vi "RSNRPZ Get Sensor Count.vi"(8 "error in (no error)":errorcluster) -> (0 "error out":errorcluster, 2 "Sensors Count":i32)   [LabVIEW 2010]
doc: "This VI returns the number of currently connected sensors."
uses:
  rsnrpz_32.dll
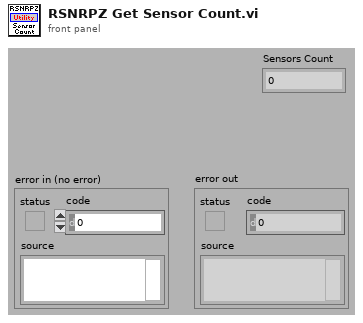
[diagram p1: front panel]
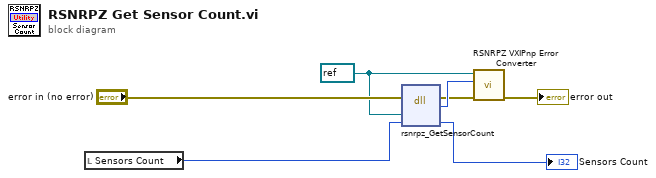
[diagram p0: block diagram]
diagram:
  w1 = refnum<visa-resource-name> refnum ("VISA session")
  n1 = local read "Sensors Count"() -> (w6:i32)
  n2 = dll-call lib="rsnrpz_32.dll" fn="rsnrpz_GetSensorCount"(error in="error in (no error)", "Instrument Handle"=w1, "Sensor Count"=w6) -> (error out=w3:errorcluster, "Status"=w7:i32, "Sensor Count"=→"Sensors Count":i32)  [unwired: 3 in, 1 out]
  n3 = call <instrlib>:"RSNRPZ VXIPnp Error Converter.vi"("error in"=w3, "VXIPnp error code"=w7, "VISA session"=w1) -> ("error out"=→"error out":errorcluster)  [unwired: 7 in, 1 out]
